vi "hw3p2_hickey.vi"() -> ()   [LabVIEW 2014]
panel:
  in  "Percent":dbl
  out "Actualy N":dbl
  out "Sum":dbl
  in  "n":i32
  in  "X":dbl
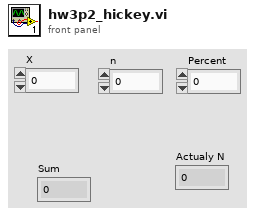
[diagram p1: front panel]
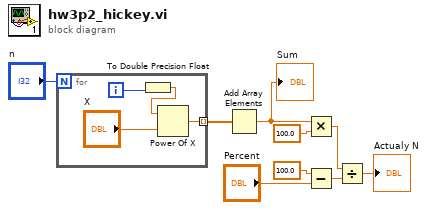
[diagram p0: block diagram]
diagram:
  n1 = for {
    N: "n" -> [_]
    tunnel: [w12] -> w8 mode=indexing
    i -> [w11]
    n2 = To Double Precision Float(number=w11) -> (double precision float=w10:dbl)
    n3 = Power Of X(1:"X", 2:w10) -> (0:w12:dbl)
  }
  n4 = Add Array Elements(numeric array=w8) -> (sum=w6:dbl)
  "Sum" <- w6
  n5 = Multiply(x=w6, y=100.0) -> (x*y=w5:dbl)
  n6 = Subtract(x=100.0, y="Percent") -> (x-y=w2:dbl)
  n7 = Divide(x=w5, y=w2) -> (x/y=→"Actualy N":dbl)
